vi "DataTXTFileRichInfo.vi"(9 "Language":u32, 11 "file path (dialog if empty)":path caption="文件路径 （空时为对话框）") -> (0 "路径输出":path, 1 "FileInfo":string, 2 "文件类型":string)   [LabVIEW 2015]
uses:
  <vilib>/regexp/Match Regular Expression.xnode
panel:
  out "匹配子字符串":string
  out "输出 2":string
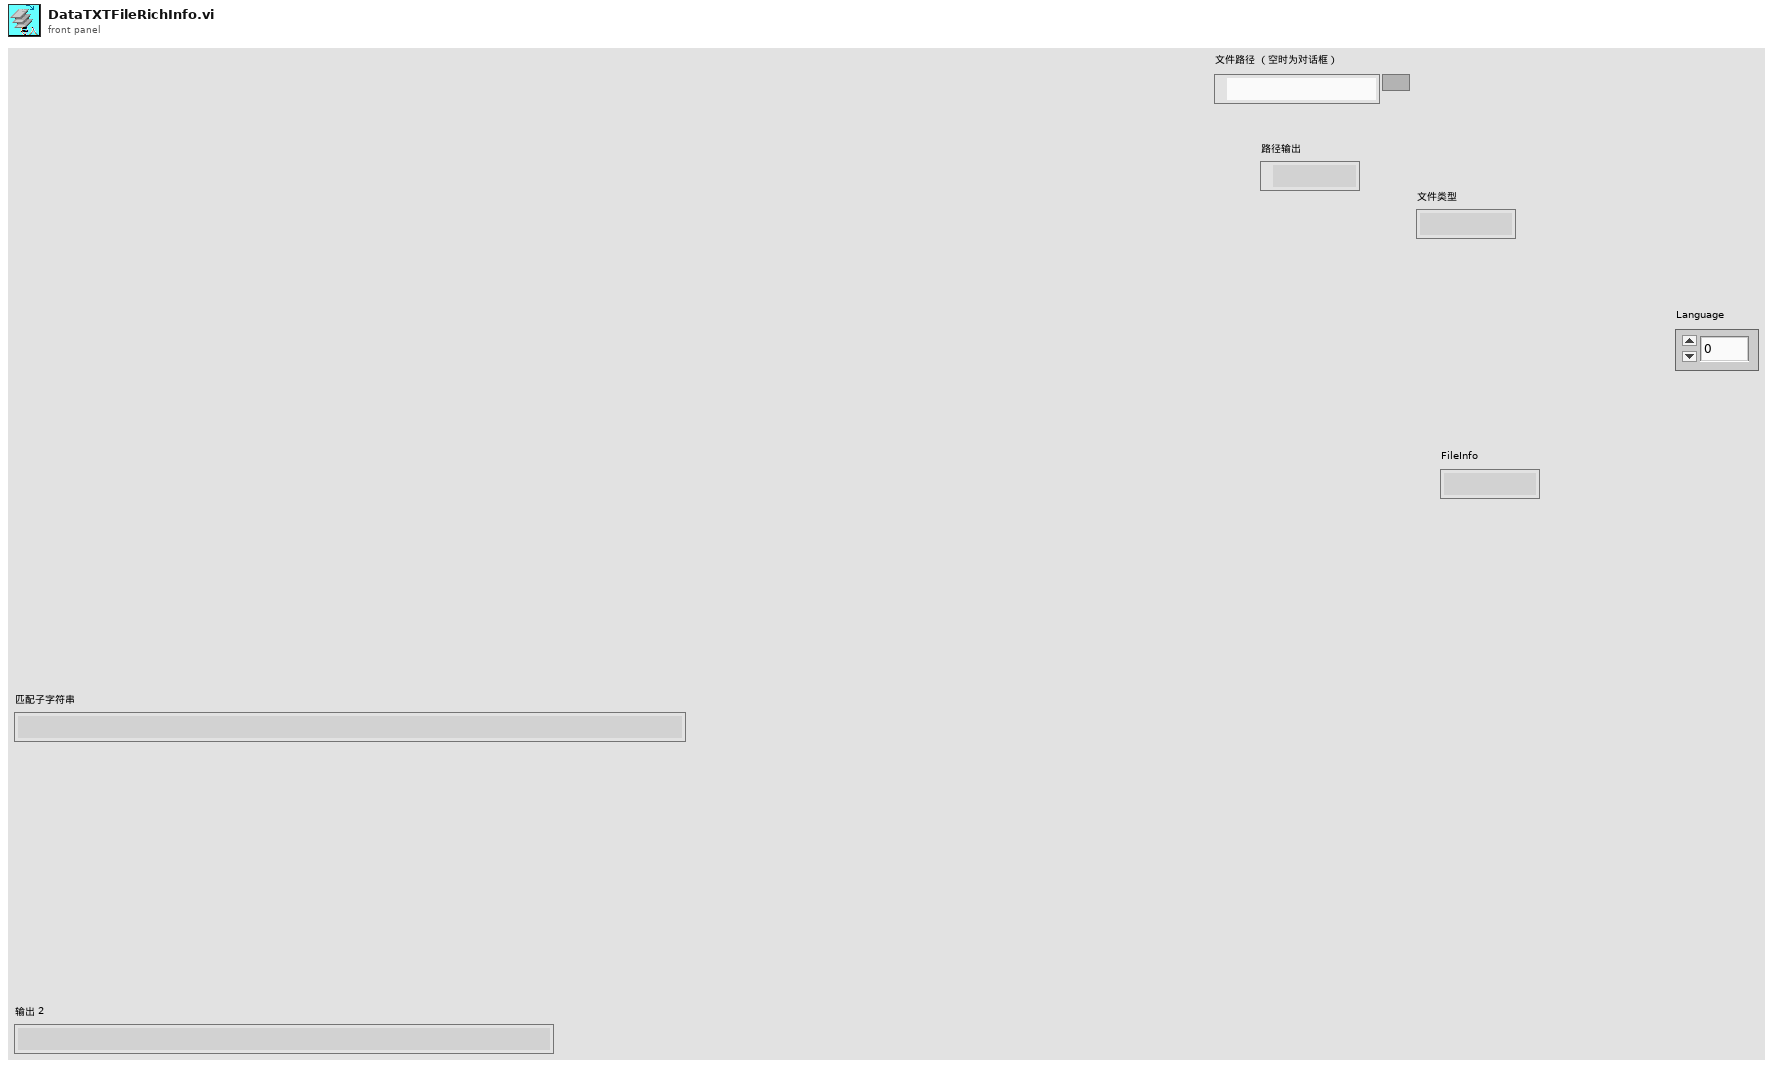
[diagram p1: front panel]
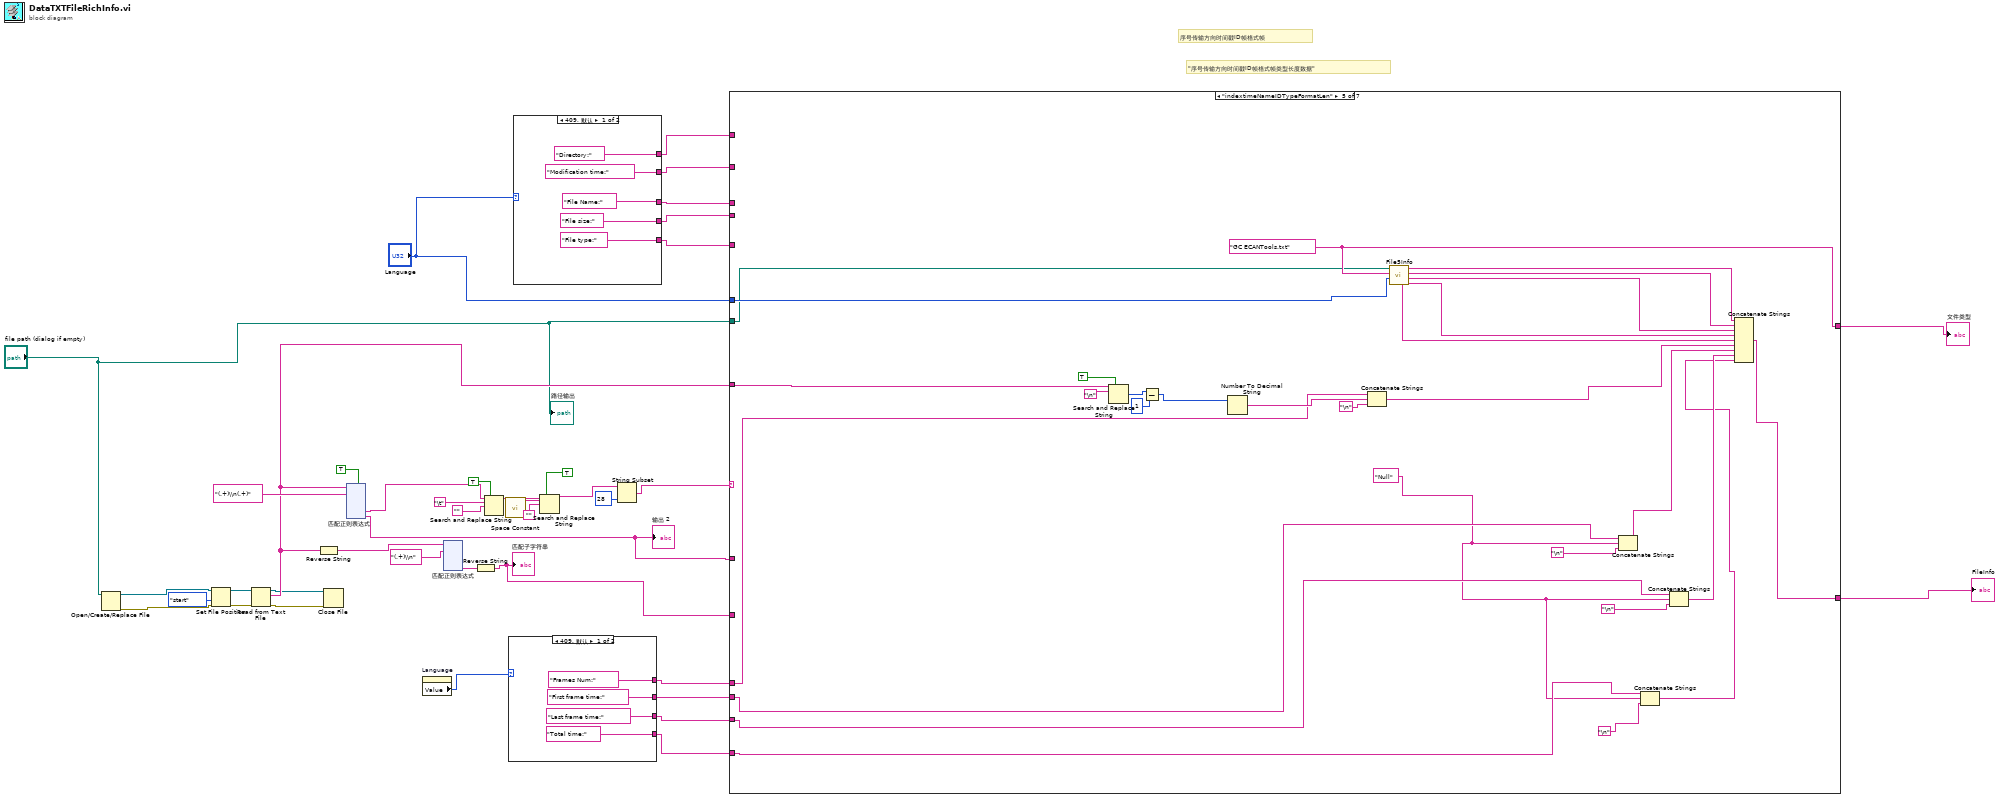
[diagram p0: block diagram]
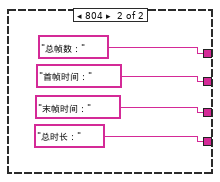
[diagram p2: hidden frame]
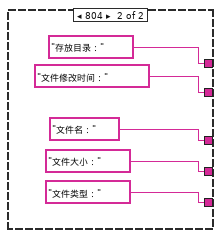
[diagram p3: hidden frame]
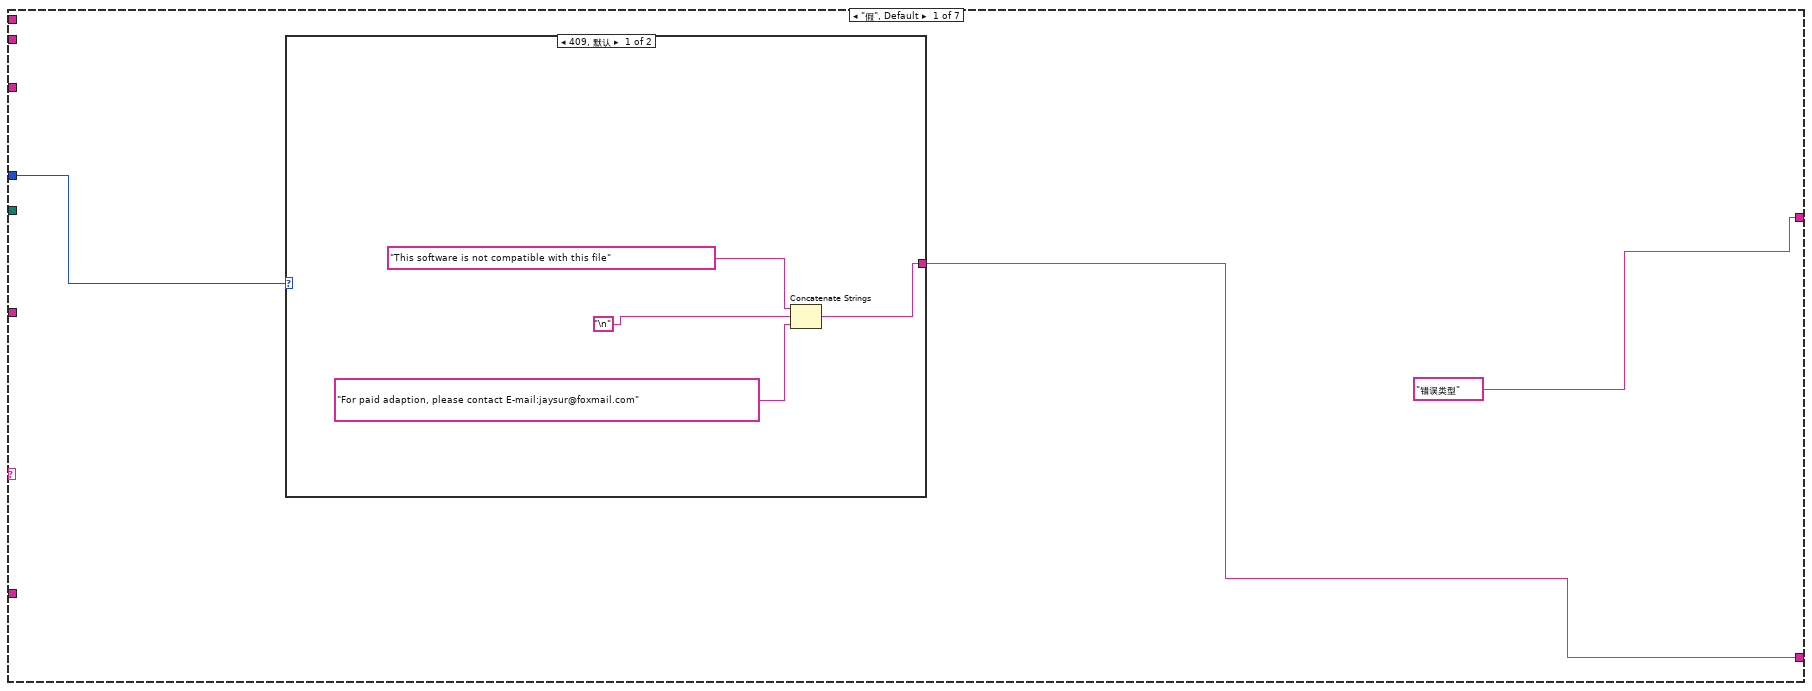
[diagram p4: hidden frame]
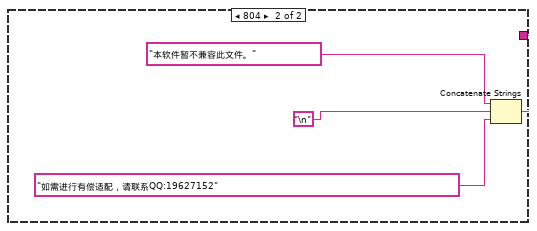
[diagram p5: hidden frame]
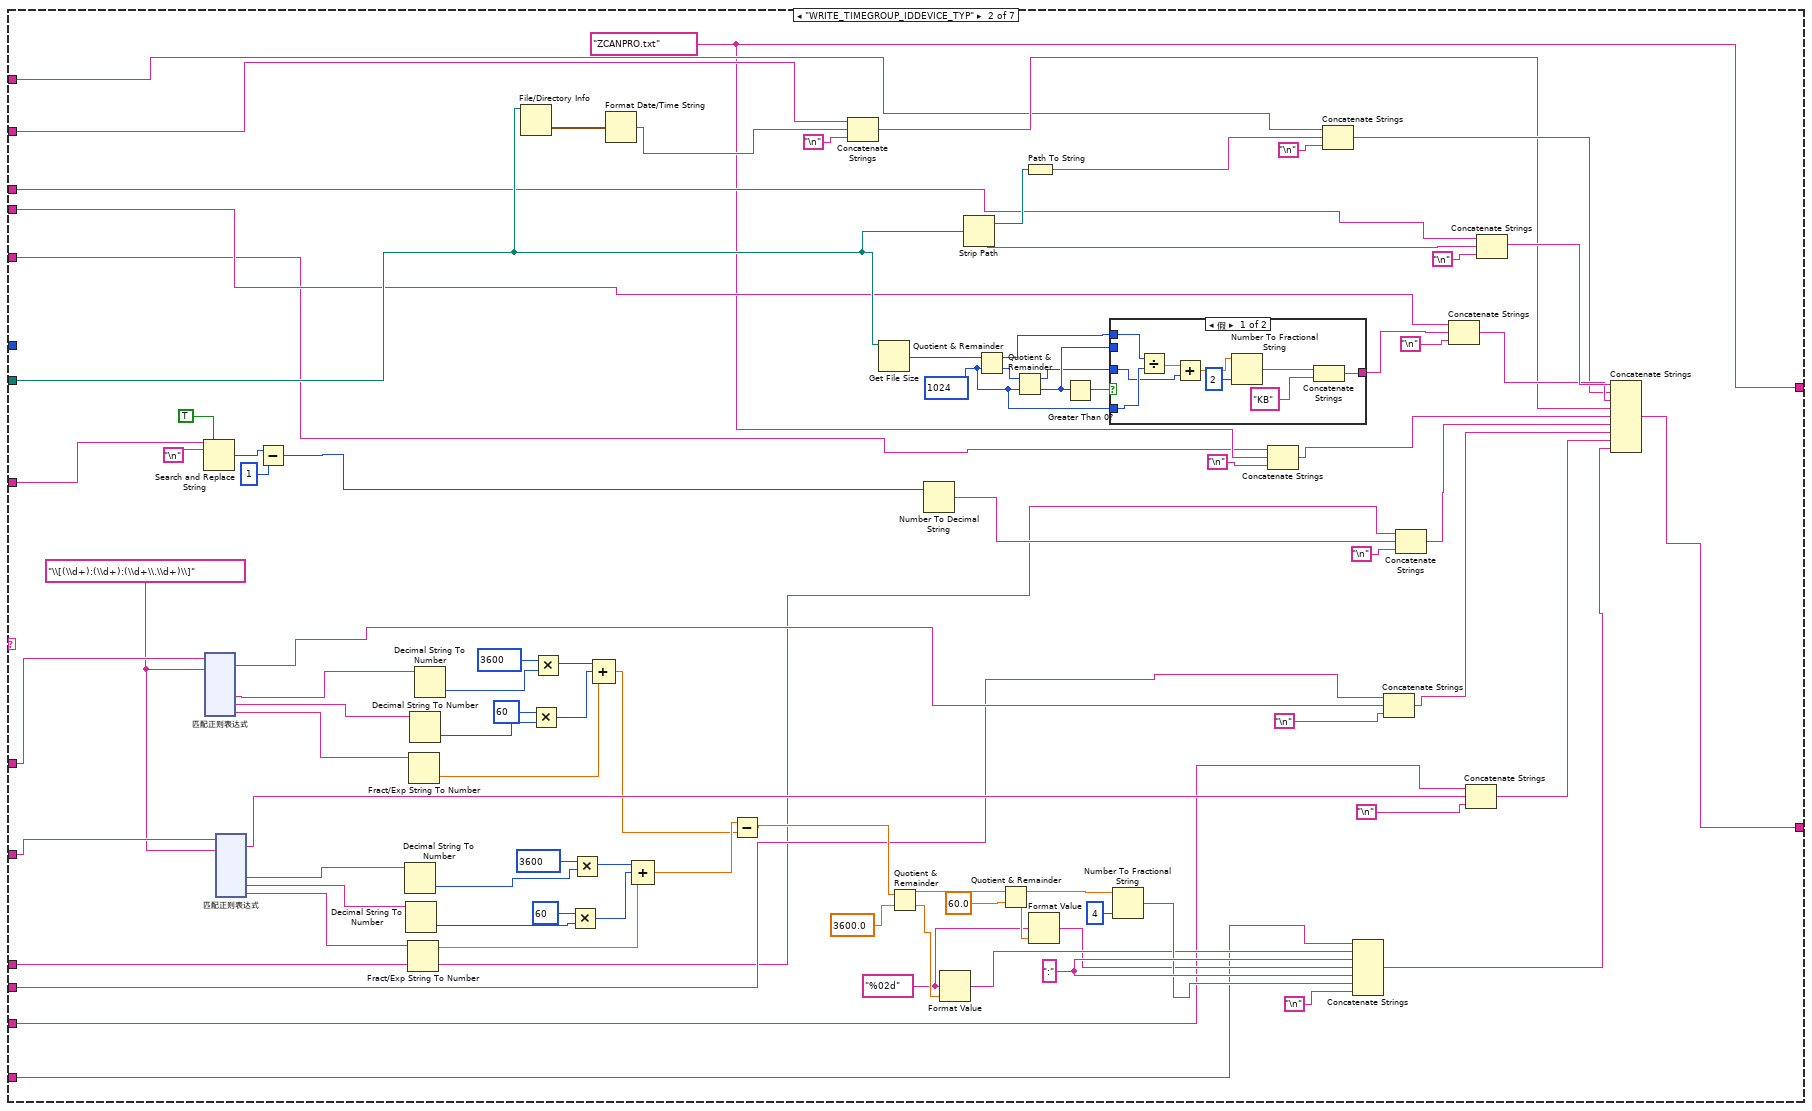
[diagram p6: hidden frame]
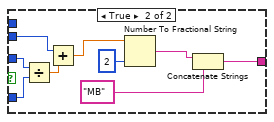
[diagram p7: hidden frame]
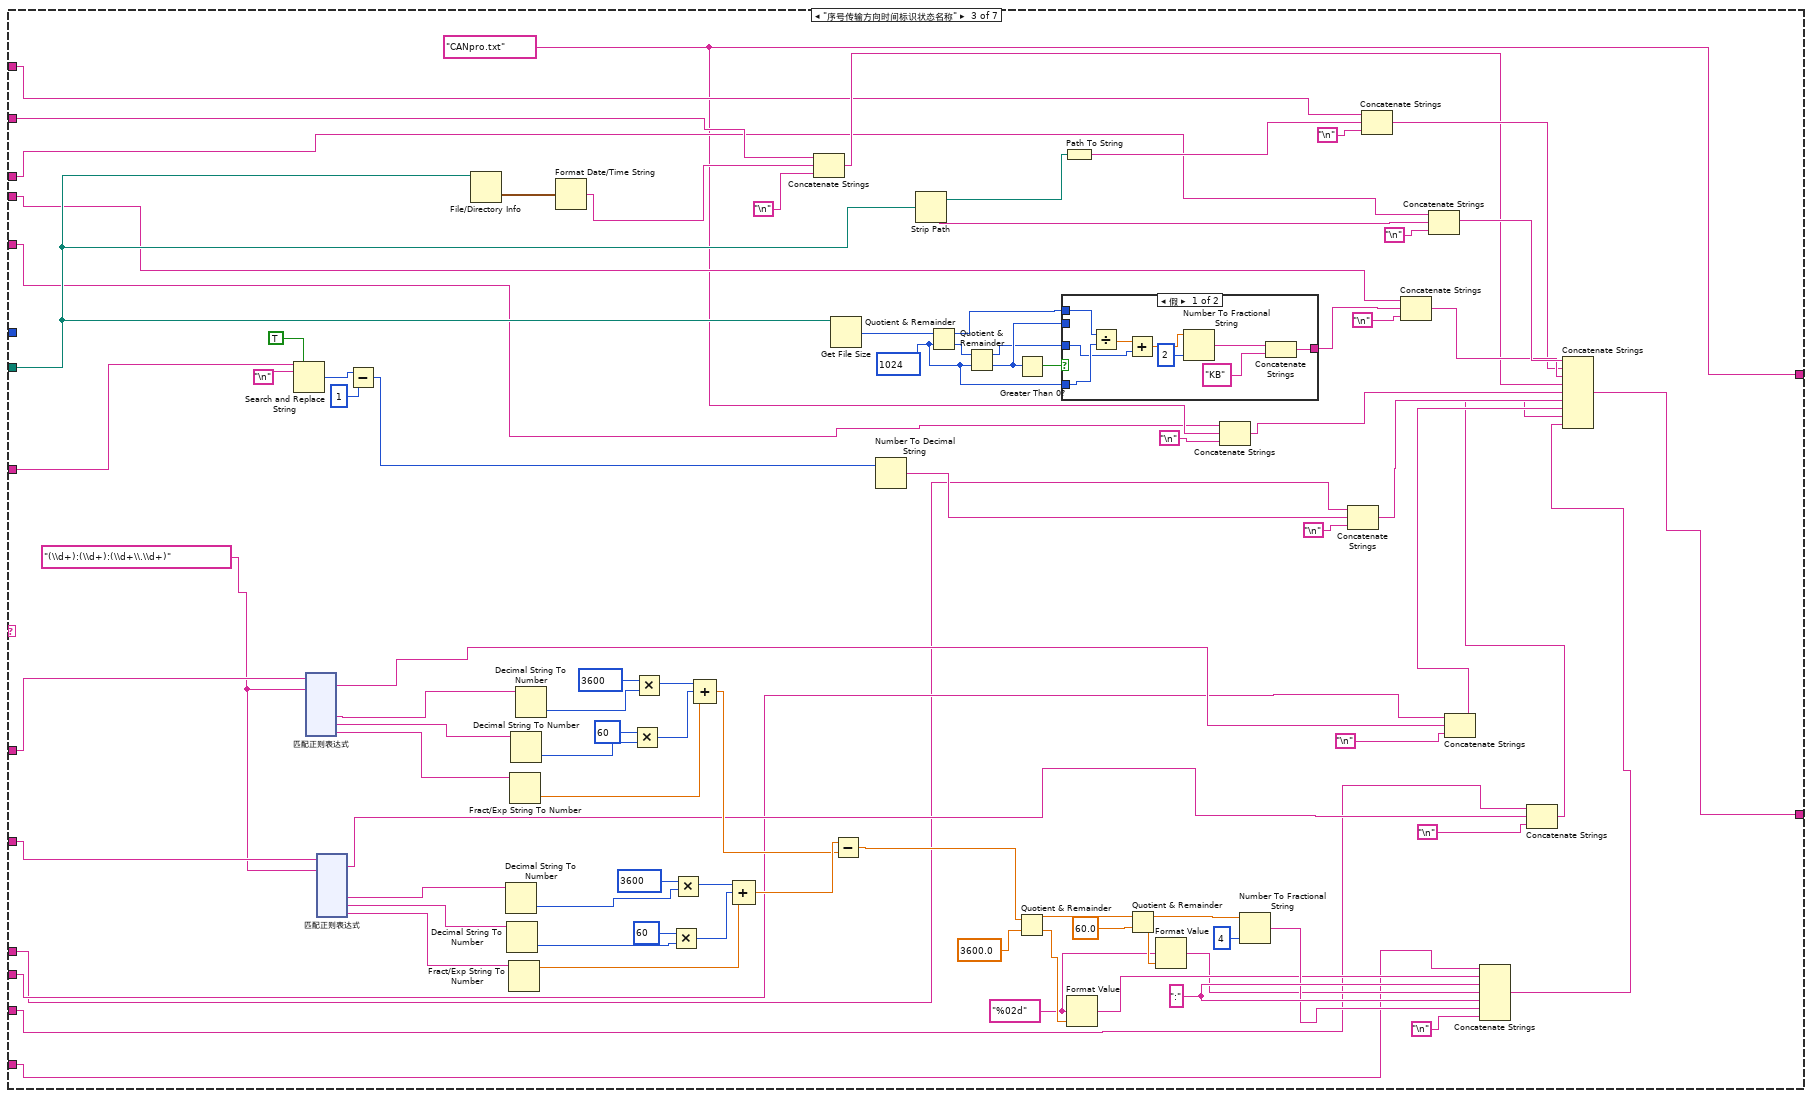
[diagram p8: hidden frame]
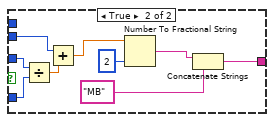
[diagram p9: hidden frame]
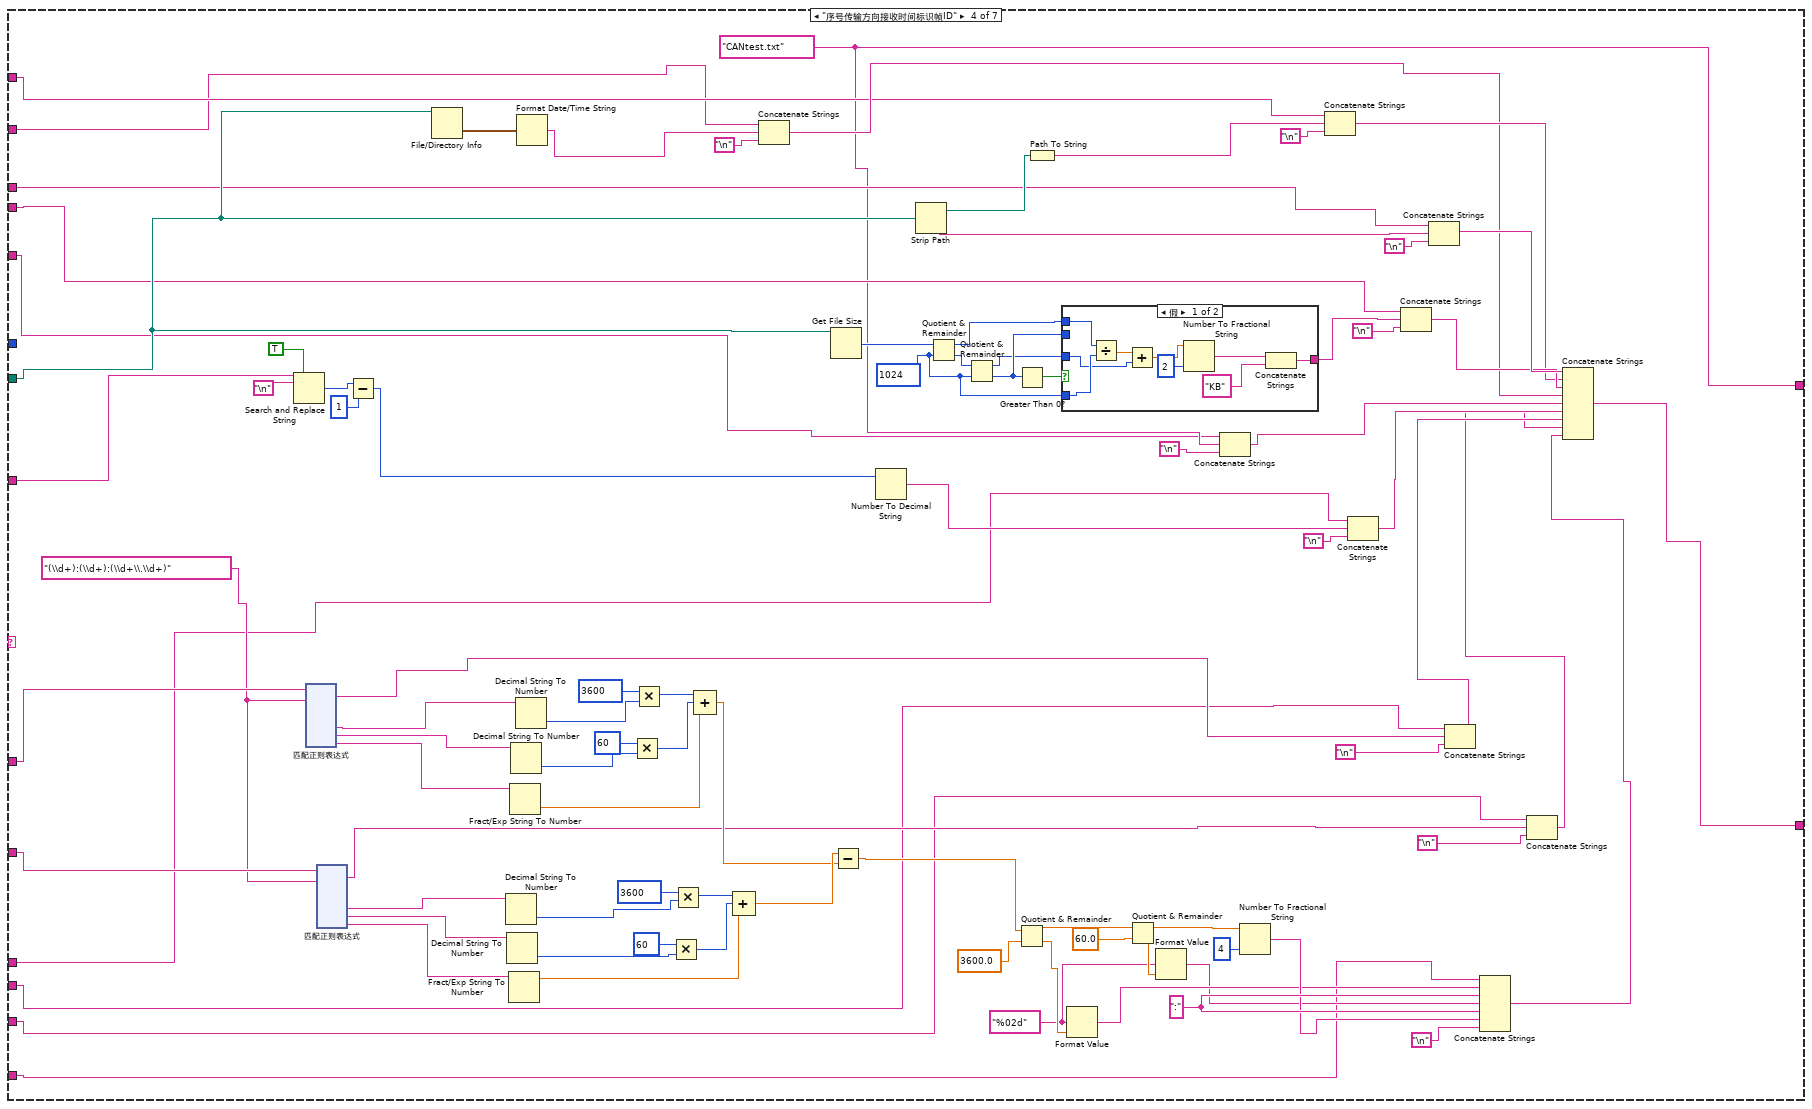
[diagram p10: hidden frame]
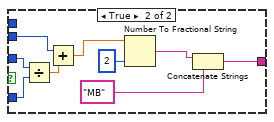
[diagram p11: hidden frame]
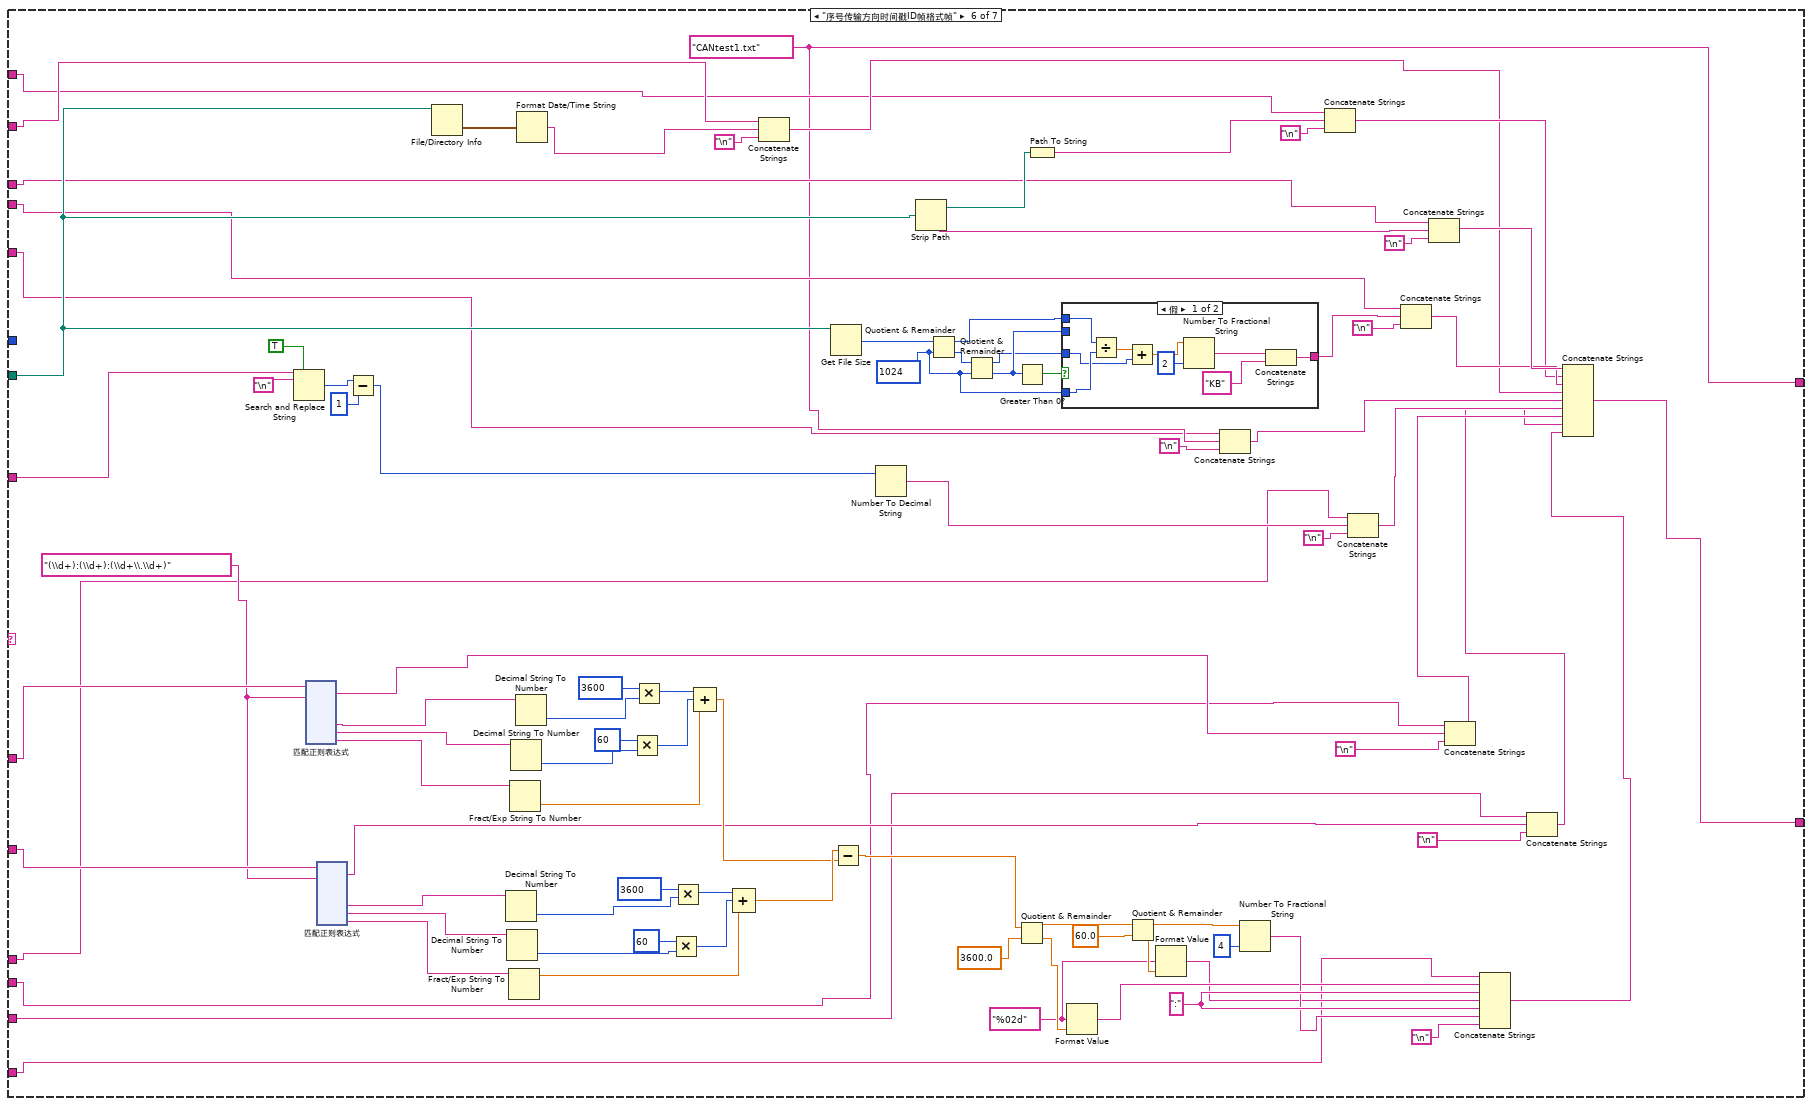
[diagram p12: hidden frame]
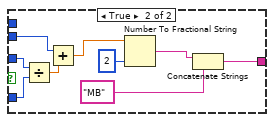
[diagram p13: hidden frame]
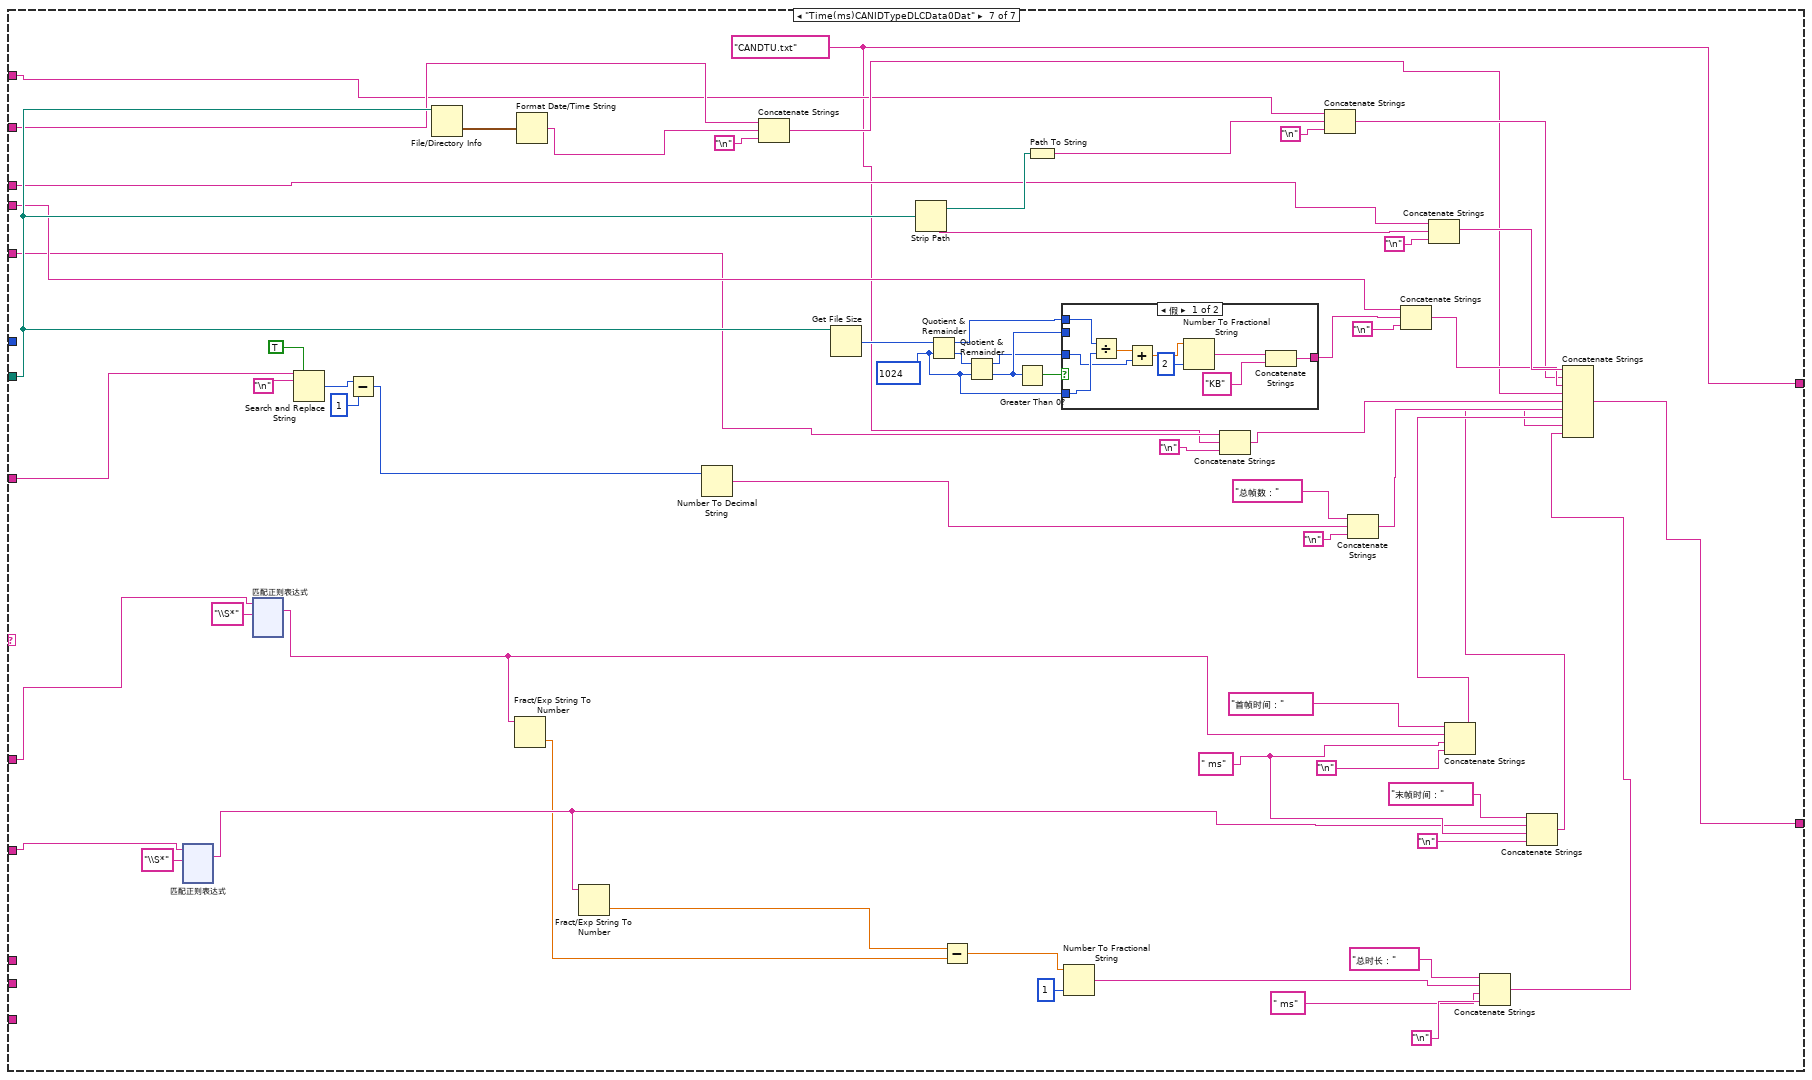
[diagram p14: hidden frame]
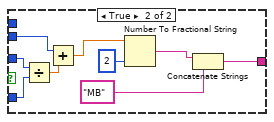
[diagram p15: hidden frame]
diagram:
  # "序号传输方向时间戳ID帧格式帧"
  # "\"序号传输方向时间戳ID帧格式帧类型长度数据\""
  n1 = Open/Create/Replace File(file path (use dialog)="file path (dialog if empty)") -> (refnum out=w17:refnum<file>, error out=w16:errorcluster)  [unwired: 5 in, 1 out]
  n2 = Set File Position(refnum=w17, from (0:start)=enum16{"start", "end", "current"}."start" ("自（0:起始）"), error in=w16) -> (refnum out=w38:refnum<file>, error out=w36:errorcluster)  [unwired: 1 in]
  n3 = Read from Text File(file (use dialog)=w38, error in=w36) -> (refnum out=w14:refnum<file>, text=w20:string, error out=w15:errorcluster)  [unwired: 2 in, 1 out]
  n4 = Reverse String(1:w20) -> (0:w24:string)
  n5 = Close File(refnum=w14, error in=w15) -> ()  [unwired: 2 out]
  n6 = xnode "匹配正则表达式"("输入字符串"=w20, "正则表达式"="(.+)\\n(.+)", "多行？(F)"=TRUE) -> ("子匹配 1"=w31:string, "子匹配 2"=w18:string)  [unwired: 3 in, 5 out]
  "输出 2" <- w18
  n7 = property on="Language" class="DigNum (严格)"() -> ("Value"=w10:u32)  [unwired: 2 in, 2 out]
  n8 = xnode "匹配正则表达式"("输入字符串"=w24, "正则表达式"="(.+)\\n") -> ("子匹配 1"=w23:string)  [unwired: 4 in, 5 out]
  n9 = Reverse String(1:w23) -> (0:w12:string)
  "匹配子字符串" <- w12
  n10 = Search and Replace String(replace all?=TRUE ("替换全部？(F)"), input string=w31, search string="\t", replace string="") -> (result string=w29:string)  [unwired: 4 in, 3 out]
  n11 = call <vilib>:"Space Constant.vi"() -> ("String"=w28:string)
  n12 = case shown="409, 默认" w10 {
    tunnel: ["Total time:" "总时长："] -> w1
    tunnel: ["Last frame time:" "末帧时间："] -> w4
    tunnel: ["First frame time:" "首帧时间："] -> w3
    tunnel: ["Frames Num:" "总帧数："] -> w2
    frame 409, Default {
    }
    frame 804 {
    }
  }
  n13 = case shown="409, 默认" "Language" {
    tunnel: ["Modification time:" "文件修改时间："] -> w9
    tunnel: ["Directory:" "存放目录："] -> w8
    tunnel: ["File Name:" "文件名："] -> w7
    tunnel: ["File size:" "文件大小："] -> w6
    tunnel: ["File type:" "文件类型："] -> w5
    frame 409, Default {
    }
    frame 804 {
    }
  }
  n14 = Search and Replace String(replace all?=TRUE ("替换全部？(F)"), input string=w29, search string=w28, replace string="") -> (result string=w22:string)  [unwired: 4 in, 3 out]
  n15 = String Subset(string=w22, length (rest)=28 ("长度（剩余）")) -> (substring=w19:string)  [unwired: 1 in]
  n16 = case shown="\"indextimeNameIDTypeFormatLen\"" w19 {
    tunnel: [w60 w126 w467 w811 w1119 w1184 w1509] -> w40
    tunnel: ["错误类型" w75 w419 w763 w1105 w1136 w1475] -> w39
    tunnel: "file path (dialog if empty)" -> [_ w81 w425 w768 w1104 w1141 w1494]
    tunnel: w20 -> [_ w118 w462 w806 w1114 w1179 w1504]
    tunnel: w18 -> [_ w114 w438 w782 _ w1155 w1492]
    tunnel: w12 -> [_ w116 w437 w781 _ w1154 w1490]
    tunnel: "Language" -> [w59 _ _ _ w1106 _ _]
    tunnel: w9 -> [_ w79 w423 w766 _ w1140 w1480]
    tunnel: w8 -> [_ w78 w422 w767 _ w1139 w1479]
    tunnel: w7 -> [_ w77 w421 w765 _ w1138 w1478]
    tunnel: w6 -> [_ w76 w420 w764 _ w1137 w1477]
    tunnel: w5 -> [_ w74 w418 w762 _ w1135 w1476]
    tunnel: w1 -> [_ w73 w417 w761 w1110 w1134 _]
    tunnel: w4 -> [_ w72 w416 w760 w1109 w1133 _]
    tunnel: w3 -> [_ w71 w415 w759 w1108 w1132 _]
    tunnel: w2 -> [_ w70 w414 w758 w1107 w1131 _]
    frame "假", Default {
      n17 = case shown="409, 默认" w59 {
        tunnel: [w62 w66] -> w60
        frame 409, Default {
          n18 = Concatenate Strings("This software is not compatible with this file", "\n", "For paid adaption, please contact E-mail:jaysur@foxmail.com") -> (w62:string)
        }
        frame 804 {
          n19 = Concatenate Strings("本软件暂不兼容此文件。", "\n", "如需进行有偿适配，请联系QQ:19627152") -> (w66:string)
        }
      }
    }
    frame "WRITE_TIMEGROUP_IDDEVICE_TYP" {
      w113 = "\\[(\\d+):(\\d+):(\\d+\\.\\d+)\\]"
      w131 = i64 1024 ("y")
      w148 = "%02d" ("格式字符串")
      w154 = ":"
      w75 = "ZCANPRO.txt"
      n20 = Search and Replace String(replace all?=TRUE ("替换全部？(F)"), input string=w118, search string="\n") -> (number of replacements=w120:i32)  [unwired: 5 in, 3 out]
      n21 = xnode "匹配正则表达式"("输入字符串"=w114, "正则表达式"=w113) -> ("所有匹配"=w112:string, "子匹配 1"=w111:string, "子匹配 2"=w110:string, "子匹配 3"=w109:string)  [unwired: 4 in, 4 out]
      n22 = xnode "匹配正则表达式"("输入字符串"=w116, "正则表达式"=w113) -> ("所有匹配"=w115:string, "子匹配 1"=w108:string, "子匹配 2"=w107:string, "子匹配 3"=w106:string)  [unwired: 4 in, 4 out]
      n23 = Subtract(x=w120, y=1) -> (x-y=w117:i32)
      n24 = Decimal String To Number(string=w108) -> (number=w94:i32)  [unwired: 2 in, 1 out]
      n25 = Decimal String To Number(string=w107) -> (number=w93:i32)  [unwired: 2 in, 1 out]
      n26 = Fract/Exp String To Number(string=w106) -> (number=w92:dbl)  [unwired: 3 in, 1 out]
      n27 = Fract/Exp String To Number(string=w109) -> (number=w99:dbl)  [unwired: 3 in, 1 out]
      n28 = Decimal String To Number(string=w110) -> (number=w105:i32)  [unwired: 2 in, 1 out]
      n29 = Decimal String To Number(string=w111) -> (number=w103:i32)  [unwired: 2 in, 1 out]
      n30 = File/Directory Info(path=w81) -> (last mod=w84:timestamp)  [unwired: 1 in, 6 out]
      n31 = Multiply(x=60, y=w105) -> (x*y=w100:i32)
      n32 = Multiply(x=3600, y=w103) -> (x*y=w101:i32)
      n33 = Multiply(x=60, y=w93) -> (x*y=w95:i32)
      n34 = Multiply(x=3600, y=w94) -> (x*y=w96:i32)
      n35 = Compound Arithmetic op=ADD(w101, w100, w99) -> (w90:dbl)
      n36 = Format Date/Time String(seconds (now)=w84) -> (date/time string=w82:string)  [unwired: 2 in]
      n37 = Compound Arithmetic op=ADD(w96, w95, w92) -> (w91:dbl)
      n38 = Subtract(x=w91, y=w90) -> (x-y=w89:dbl)
      n39 = Concatenate Strings(w79, w82, "\n") -> (w80:string)
      n40 = Get File Size(file=w81) -> (size (in bytes)=w134:i64)  [unwired: 1 in, 2 out]
      n41 = Quotient & Remainder(x=w89, y=3600.0) -> (x-y*floor(x/y)=w158:dbl, floor(x/y)=w151:dbl)
      n42 = Number To Decimal String(number=w117) -> (decimal integer string=w137:string)  [unwired: 1 in]
      n43 = Format Value(format string=w148, value (0)=w151) -> (output string=w152:string)  [unwired: 1 in]
      n44 = Strip Path(path=w81) -> (stripped path=w86:path, name=w144:string)
      n45 = Quotient & Remainder(x=w134, y=w131) -> (x-y*floor(x/y)=w127:i64, floor(x/y)=w133:i64)
      n46 = Quotient & Remainder(x=w158, y=60.0) -> (x-y*floor(x/y)=w156:dbl, floor(x/y)=w150:dbl)
      n47 = Quotient & Remainder(x=w133, y=w131) -> (x-y*floor(x/y)=w129:i64, floor(x/y)=w130:i64)
      n48 = Path To String(path=w86) -> (string=w87:string)
      n49 = Format Value(format string=w148, value (0)=w150) -> (output string=w149:string)  [unwired: 1 in]
      n50 = Greater Than 0?(x=w130) -> (x > 0?=w132:bool)
      n51 = case shown="假" w132 {
        tunnel: w131 -> [w401 w411]
        tunnel: w130 -> [_ w409]
        tunnel: w129 -> [w399 w412]
        tunnel: [w404 w407] -> w128
        tunnel: w127 -> [w402 _]
        frame False {
          n52 = Divide(x=w402, y=w401) -> (x/y=w400:dbl)
          n53 = Add(x=w400, y=w399) -> (x+y=w398:dbl)
          n54 = Number To Fractional String(number=w398, precision (6)=i16 2 ("精度(6)")) -> (F-format string=w396:string)  [unwired: 2 in]
          n55 = Concatenate Strings(w396, "KB" ("字符串")) -> (w404:string)
        }
        frame True {
          n56 = Divide(x=w412, y=w411) -> (x/y=w410:dbl)
          n57 = Add(x=w409, y=w410) -> (x+y=w408:dbl)
          n58 = Number To Fractional String(number=w408, precision (6)=i16 2 ("精度(6)")) -> (F-format string=w406:string)  [unwired: 2 in]
          n59 = Concatenate Strings(w406, "MB") -> (w407:string)
        }
      }
      n60 = Number To Fractional String(number=w156, precision (6)=i16 4 ("精度(6)")) -> (F-format string=w153:string)  [unwired: 2 in]
      n61 = Concatenate Strings(w74, w75, "\n") -> (w141:string)
      n62 = Concatenate Strings(w78, w87, "\n") -> (w85:string)
      n63 = Concatenate Strings(w73, w152, w154, w149, w154, w153, "\n") -> (w125:string)
      n64 = Concatenate Strings(w71, w112, "\n") -> (w123:string)
      n65 = Concatenate Strings(w70, w137, "\n") -> (w138:string)
      n66 = Concatenate Strings(w76, w128, "\n") -> (w135:string)
      n67 = Concatenate Strings(w72, w115, "\n") -> (w124:string)
      n68 = Concatenate Strings(w77, w144, "\n") -> (w143:string)
      n69 = Concatenate Strings(w143, w85, w135, w80, w141, w138, w123, w124, w125) -> (w126:string)
    }
    frame "序号传输方向时间标识状态名称" {
      w434 = "(\\d+):(\\d+):(\\d+\\.\\d+)"
      w475 = i64 1024 ("y")
      w492 = "%02d" ("格式字符串")
      w498 = ":"
      w419 = "CANpro.txt"
      n70 = Search and Replace String(replace all?=TRUE ("替换全部？(F)"), input string=w462, search string="\n") -> (number of replacements=w464:i32)  [unwired: 5 in, 3 out]
      n71 = xnode "匹配正则表达式"("输入字符串"=w438, "正则表达式"=w434) -> ("所有匹配"=w436:string, "子匹配 1"=w460:string, "子匹配 2"=w459:string, "子匹配 3"=w458:string)  [unwired: 4 in, 4 out]
      n72 = xnode "匹配正则表达式"("输入字符串"=w437, "正则表达式"=w434) -> ("所有匹配"=w435:string, "子匹配 1"=w457:string, "子匹配 2"=w456:string, "子匹配 3"=w455:string)  [unwired: 4 in, 4 out]
      n73 = Subtract(x=w464, y=1) -> (x-y=w461:i32)
      n74 = File/Directory Info(path=w425) -> (last mod=w428:timestamp)  [unwired: 1 in, 6 out]
      n75 = Decimal String To Number(string=w457) -> (number=w443:i32)  [unwired: 2 in, 1 out]
      n76 = Decimal String To Number(string=w456) -> (number=w442:i32)  [unwired: 2 in, 1 out]
      n77 = Fract/Exp String To Number(string=w455) -> (number=w441:dbl)  [unwired: 3 in, 1 out]
      n78 = Fract/Exp String To Number(string=w458) -> (number=w448:dbl)  [unwired: 3 in, 1 out]
      n79 = Decimal String To Number(string=w459) -> (number=w454:i32)  [unwired: 2 in, 1 out]
      n80 = Decimal String To Number(string=w460) -> (number=w452:i32)  [unwired: 2 in, 1 out]
      n81 = Format Date/Time String(seconds (now)=w428) -> (date/time string=w426:string)  [unwired: 2 in]
      n82 = Multiply(x=60, y=w454) -> (x*y=w449:i32)
      n83 = Multiply(x=3600, y=w452) -> (x*y=w450:i32)
      n84 = Multiply(x=60, y=w442) -> (x*y=w444:i32)
      n85 = Multiply(x=3600, y=w443) -> (x*y=w445:i32)
      n86 = Compound Arithmetic op=ADD(w450, w449, w448) -> (w439:dbl)
      n87 = Compound Arithmetic op=ADD(w445, w444, w441) -> (w440:dbl)
      n88 = Concatenate Strings(w423, w426, "\n") -> (w424:string)
      n89 = Get File Size(file=w425) -> (size (in bytes)=w478:i64)  [unwired: 1 in, 2 out]
      n90 = Subtract(x=w440, y=w439) -> (x-y=w433:dbl)
      n91 = Number To Decimal String(number=w461) -> (decimal integer string=w481:string)  [unwired: 1 in]
      n92 = Strip Path(path=w425) -> (stripped path=w430:path, name=w488:string)
      n93 = Quotient & Remainder(x=w478, y=w475) -> (x-y*floor(x/y)=w471:i64, floor(x/y)=w477:i64)
      n94 = Quotient & Remainder(x=w477, y=w475) -> (x-y*floor(x/y)=w473:i64, floor(x/y)=w474:i64)
      n95 = Greater Than 0?(x=w474) -> (x > 0?=w476:bool)
      n96 = Quotient & Remainder(x=w433, y=3600.0) -> (x-y*floor(x/y)=w502:dbl, floor(x/y)=w495:dbl)
      n97 = case shown="假" w476 {
        tunnel: w475 -> [w745 w755]
        tunnel: w474 -> [_ w753]
        tunnel: w473 -> [w743 w756]
        tunnel: [w748 w751] -> w472
        tunnel: w471 -> [w746 _]
        frame False {
          n98 = Divide(x=w746, y=w745) -> (x/y=w744:dbl)
          n99 = Add(x=w744, y=w743) -> (x+y=w742:dbl)
          n100 = Number To Fractional String(number=w742, precision (6)=i16 2 ("精度(6)")) -> (F-format string=w740:string)  [unwired: 2 in]
          n101 = Concatenate Strings(w740, "KB" ("字符串")) -> (w748:string)
        }
        frame True {
          n102 = Divide(x=w756, y=w755) -> (x/y=w754:dbl)
          n103 = Add(x=w753, y=w754) -> (x+y=w752:dbl)
          n104 = Number To Fractional String(number=w752, precision (6)=i16 2 ("精度(6)")) -> (F-format string=w750:string)  [unwired: 2 in]
          n105 = Concatenate Strings(w750, "MB") -> (w751:string)
        }
      }
      n106 = Path To String(path=w430) -> (string=w431:string)
      n107 = Format Value(format string=w492, value (0)=w495) -> (output string=w496:string)  [unwired: 1 in]
      n108 = Quotient & Remainder(x=w502, y=60.0) -> (x-y*floor(x/y)=w500:dbl, floor(x/y)=w494:dbl)
      n109 = Format Value(format string=w492, value (0)=w494) -> (output string=w493:string)  [unwired: 1 in]
      n110 = Concatenate Strings(w418, w419, "\n") -> (w485:string)
      n111 = Number To Fractional String(number=w500, precision (6)=i16 4 ("精度(6)")) -> (F-format string=w497:string)  [unwired: 2 in]
      n112 = Concatenate Strings(w414, w481, "\n") -> (w482:string)
      n113 = Concatenate Strings(w422, w431, "\n") -> (w429:string)
      n114 = Concatenate Strings(w420, w472, "\n") -> (w479:string)
      n115 = Concatenate Strings(w421, w488, "\n") -> (w487:string)
      n116 = Concatenate Strings(w415, w436, "\n") -> (w470:string)
      n117 = Concatenate Strings(w417, w496, w498, w493, w498, w497, "\n") -> (w468:string)
      n118 = Concatenate Strings(w416, w435, "\n") -> (w469:string)
      n119 = Concatenate Strings(w487, w429, w479, w424, w485, w482, w470, w469, w468) -> (w467:string)
    }
    frame "序号传输方向接收时间标识帧ID" {
      w778 = "(\\d+):(\\d+):(\\d+\\.\\d+)"
      w819 = i64 1024 ("y")
      w836 = "%02d" ("格式字符串")
      w842 = ":"
      w763 = "CANtest.txt"
      n120 = Search and Replace String(replace all?=TRUE ("替换全部？(F)"), input string=w806, search string="\n") -> (number of replacements=w808:i32)  [unwired: 5 in, 3 out]
      n121 = xnode "匹配正则表达式"("输入字符串"=w782, "正则表达式"=w778) -> ("所有匹配"=w780:string, "子匹配 1"=w804:string, "子匹配 2"=w803:string, "子匹配 3"=w802:string)  [unwired: 4 in, 4 out]
      n122 = xnode "匹配正则表达式"("输入字符串"=w781, "正则表达式"=w778) -> ("所有匹配"=w779:string, "子匹配 1"=w801:string, "子匹配 2"=w800:string, "子匹配 3"=w799:string)  [unwired: 4 in, 4 out]
      n123 = Subtract(x=w808, y=1) -> (x-y=w805:i32)
      n124 = File/Directory Info(path=w768) -> (last mod=w772:timestamp)  [unwired: 1 in, 6 out]
      n125 = Decimal String To Number(string=w801) -> (number=w787:i32)  [unwired: 2 in, 1 out]
      n126 = Decimal String To Number(string=w800) -> (number=w786:i32)  [unwired: 2 in, 1 out]
      n127 = Fract/Exp String To Number(string=w799) -> (number=w785:dbl)  [unwired: 3 in, 1 out]
      n128 = Fract/Exp String To Number(string=w802) -> (number=w792:dbl)  [unwired: 3 in, 1 out]
      n129 = Decimal String To Number(string=w803) -> (number=w798:i32)  [unwired: 2 in, 1 out]
      n130 = Decimal String To Number(string=w804) -> (number=w796:i32)  [unwired: 2 in, 1 out]
      n131 = Format Date/Time String(seconds (now)=w772) -> (date/time string=w770:string)  [unwired: 2 in]
      n132 = Multiply(x=60, y=w798) -> (x*y=w793:i32)
      n133 = Multiply(x=3600, y=w796) -> (x*y=w794:i32)
      n134 = Multiply(x=60, y=w786) -> (x*y=w788:i32)
      n135 = Multiply(x=3600, y=w787) -> (x*y=w789:i32)
      n136 = Compound Arithmetic op=ADD(w794, w793, w792) -> (w783:dbl)
      n137 = Compound Arithmetic op=ADD(w789, w788, w785) -> (w784:dbl)
      n138 = Concatenate Strings(w766, w770, "\n") -> (w769:string)
      n139 = Get File Size(file=w768) -> (size (in bytes)=w822:i64)  [unwired: 1 in, 2 out]
      n140 = Subtract(x=w784, y=w783) -> (x-y=w777:dbl)
      n141 = Number To Decimal String(number=w805) -> (decimal integer string=w825:string)  [unwired: 1 in]
      n142 = Strip Path(path=w768) -> (stripped path=w774:path, name=w832:string)
      n143 = Quotient & Remainder(x=w822, y=w819) -> (x-y*floor(x/y)=w815:i64, floor(x/y)=w821:i64)
      n144 = Quotient & Remainder(x=w821, y=w819) -> (x-y*floor(x/y)=w817:i64, floor(x/y)=w818:i64)
      n145 = Greater Than 0?(x=w818) -> (x > 0?=w820:bool)
      n146 = Quotient & Remainder(x=w777, y=3600.0) -> (x-y*floor(x/y)=w846:dbl, floor(x/y)=w839:dbl)
      n147 = Path To String(path=w774) -> (string=w775:string)
      n148 = case shown="假" w820 {
        tunnel: w819 -> [w1089 w1099]
        tunnel: w818 -> [_ w1097]
        tunnel: w817 -> [w1087 w1100]
        tunnel: [w1092 w1095] -> w816
        tunnel: w815 -> [w1090 _]
        frame False {
          n149 = Divide(x=w1090, y=w1089) -> (x/y=w1088:dbl)
          n150 = Add(x=w1088, y=w1087) -> (x+y=w1086:dbl)
          n151 = Number To Fractional String(number=w1086, precision (6)=i16 2 ("精度(6)")) -> (F-format string=w1084:string)  [unwired: 2 in]
          n152 = Concatenate Strings(w1084, "KB" ("字符串")) -> (w1092:string)
        }
        frame True {
          n153 = Divide(x=w1100, y=w1099) -> (x/y=w1098:dbl)
          n154 = Add(x=w1097, y=w1098) -> (x+y=w1096:dbl)
          n155 = Number To Fractional String(number=w1096, precision (6)=i16 2 ("精度(6)")) -> (F-format string=w1094:string)  [unwired: 2 in]
          n156 = Concatenate Strings(w1094, "MB") -> (w1095:string)
        }
      }
      n157 = Format Value(format string=w836, value (0)=w839) -> (output string=w840:string)  [unwired: 1 in]
      n158 = Quotient & Remainder(x=w846, y=60.0) -> (x-y*floor(x/y)=w844:dbl, floor(x/y)=w838:dbl)
      n159 = Format Value(format string=w836, value (0)=w838) -> (output string=w837:string)  [unwired: 1 in]
      n160 = Concatenate Strings(w762, w763, "\n") -> (w829:string)
      n161 = Number To Fractional String(number=w844, precision (6)=i16 4 ("精度(6)")) -> (F-format string=w841:string)  [unwired: 2 in]
      n162 = Concatenate Strings(w767, w775, "\n") -> (w773:string)
      n163 = Concatenate Strings(w758, w825, "\n") -> (w826:string)
      n164 = Concatenate Strings(w764, w816, "\n") -> (w823:string)
      n165 = Concatenate Strings(w765, w832, "\n") -> (w831:string)
      n166 = Concatenate Strings(w759, w780, "\n") -> (w814:string)
      n167 = Concatenate Strings(w761, w840, w842, w837, w842, w841, "\n") -> (w812:string)
      n168 = Concatenate Strings(w760, w779, "\n") -> (w813:string)
      n169 = Concatenate Strings(w831, w773, w823, w769, w829, w826, w814, w813, w812) -> (w811:string)
    }
    frame "indextimeNameIDTypeFormatLen" {
      w1103 = "Null"
      w1105 = "GC ECANTools.txt"
      n170 = Search and Replace String(replace all?=TRUE ("替换全部？(F)"), input string=w1114, search string="\n") -> (number of replacements=w1116:i32)  [unwired: 5 in, 3 out]
      n171 = Subtract(x=w1116, y=1) -> (x-y=w1113:i32)
      n172 = Number To Decimal String(number=w1113) -> (decimal integer string=w1124:string)  [unwired: 1 in]
      n173 = Concatenate Strings(w1107, w1124, "\n") -> (w1125:string)
      n174 = call "File5Info.vi"("Language"=w1106, "TypeIn"=w1105, "file path (dialog if empty)"=w1104) -> ("ModificationTimeOut"=w1111:string, "FileSizeOut"=w1123:string, "DirectoryOut"=w1112:string, "FileNameOut"=w1128:string, "FileTypeOut"=w1127:string)  [unwired: 4 in]
      n175 = Concatenate Strings(w1108, w1103, "\n") -> (w1122:string)
      n176 = Concatenate Strings(w1110, w1103, "\n") -> (w1120:string)
      n177 = Concatenate Strings(w1109, w1103, "\n") -> (w1121:string)
      n178 = Concatenate Strings(w1128, w1112, w1123, w1111, w1127, w1125, w1122, w1121, w1120) -> (w1119:string)
    }
    frame "序号传输方向时间戳ID帧格式帧" {
      w1151 = "(\\d+):(\\d+):(\\d+\\.\\d+)"
      w1192 = i64 1024 ("y")
      w1209 = "%02d" ("格式字符串")
      w1215 = ":"
      w1136 = "CANtest1.txt"
      n179 = Search and Replace String(replace all?=TRUE ("替换全部？(F)"), input string=w1179, search string="\n") -> (number of replacements=w1181:i32)  [unwired: 5 in, 3 out]
      n180 = xnode "匹配正则表达式"("输入字符串"=w1155, "正则表达式"=w1151) -> ("所有匹配"=w1153:string, "子匹配 1"=w1177:string, "子匹配 2"=w1176:string, "子匹配 3"=w1175:string)  [unwired: 4 in, 4 out]
      n181 = xnode "匹配正则表达式"("输入字符串"=w1154, "正则表达式"=w1151) -> ("所有匹配"=w1152:string, "子匹配 1"=w1174:string, "子匹配 2"=w1173:string, "子匹配 3"=w1172:string)  [unwired: 4 in, 4 out]
      n182 = Subtract(x=w1181, y=1) -> (x-y=w1178:i32)
      n183 = File/Directory Info(path=w1141) -> (last mod=w1145:timestamp)  [unwired: 1 in, 6 out]
      n184 = Decimal String To Number(string=w1174) -> (number=w1160:i32)  [unwired: 2 in, 1 out]
      n185 = Decimal String To Number(string=w1173) -> (number=w1159:i32)  [unwired: 2 in, 1 out]
      n186 = Fract/Exp String To Number(string=w1172) -> (number=w1158:dbl)  [unwired: 3 in, 1 out]
      n187 = Fract/Exp String To Number(string=w1175) -> (number=w1165:dbl)  [unwired: 3 in, 1 out]
      n188 = Decimal String To Number(string=w1176) -> (number=w1171:i32)  [unwired: 2 in, 1 out]
      n189 = Decimal String To Number(string=w1177) -> (number=w1169:i32)  [unwired: 2 in, 1 out]
      n190 = Format Date/Time String(seconds (now)=w1145) -> (date/time string=w1143:string)  [unwired: 2 in]
      n191 = Multiply(x=60, y=w1171) -> (x*y=w1166:i32)
      n192 = Multiply(x=3600, y=w1169) -> (x*y=w1167:i32)
      n193 = Multiply(x=60, y=w1159) -> (x*y=w1161:i32)
      n194 = Multiply(x=3600, y=w1160) -> (x*y=w1162:i32)
      n195 = Compound Arithmetic op=ADD(w1167, w1166, w1165) -> (w1156:dbl)
      n196 = Compound Arithmetic op=ADD(w1162, w1161, w1158) -> (w1157:dbl)
      n197 = Concatenate Strings(w1140, w1143, "\n") -> (w1142:string)
      n198 = Get File Size(file=w1141) -> (size (in bytes)=w1195:i64)  [unwired: 1 in, 2 out]
      n199 = Subtract(x=w1157, y=w1156) -> (x-y=w1150:dbl)
      n200 = Number To Decimal String(number=w1178) -> (decimal integer string=w1198:string)  [unwired: 1 in]
      n201 = Strip Path(path=w1141) -> (stripped path=w1147:path, name=w1205:string)
      n202 = Quotient & Remainder(x=w1195, y=w1192) -> (x-y*floor(x/y)=w1188:i64, floor(x/y)=w1194:i64)
      n203 = Quotient & Remainder(x=w1194, y=w1192) -> (x-y*floor(x/y)=w1190:i64, floor(x/y)=w1191:i64)
      n204 = Greater Than 0?(x=w1191) -> (x > 0?=w1193:bool)
      n205 = Quotient & Remainder(x=w1150, y=3600.0) -> (x-y*floor(x/y)=w1219:dbl, floor(x/y)=w1212:dbl)
      n206 = Path To String(path=w1147) -> (string=w1148:string)
      n207 = case shown="假" w1193 {
        tunnel: w1192 -> [w1462 w1472]
        tunnel: w1191 -> [_ w1470]
        tunnel: w1190 -> [w1460 w1473]
        tunnel: [w1465 w1468] -> w1189
        tunnel: w1188 -> [w1463 _]
        frame False {
          n208 = Divide(x=w1463, y=w1462) -> (x/y=w1461:dbl)
          n209 = Add(x=w1461, y=w1460) -> (x+y=w1459:dbl)
          n210 = Number To Fractional String(number=w1459, precision (6)=i16 2 ("精度(6)")) -> (F-format string=w1457:string)  [unwired: 2 in]
          n211 = Concatenate Strings(w1457, "KB" ("字符串")) -> (w1465:string)
        }
        frame True {
          n212 = Divide(x=w1473, y=w1472) -> (x/y=w1471:dbl)
          n213 = Add(x=w1470, y=w1471) -> (x+y=w1469:dbl)
          n214 = Number To Fractional String(number=w1469, precision (6)=i16 2 ("精度(6)")) -> (F-format string=w1467:string)  [unwired: 2 in]
          n215 = Concatenate Strings(w1467, "MB") -> (w1468:string)
        }
      }
      n216 = Format Value(format string=w1209, value (0)=w1212) -> (output string=w1213:string)  [unwired: 1 in]
      n217 = Quotient & Remainder(x=w1219, y=60.0) -> (x-y*floor(x/y)=w1217:dbl, floor(x/y)=w1211:dbl)
      n218 = Format Value(format string=w1209, value (0)=w1211) -> (output string=w1210:string)  [unwired: 1 in]
      n219 = Concatenate Strings(w1135, w1136, "\n") -> (w1202:string)
      n220 = Number To Fractional String(number=w1217, precision (6)=i16 4 ("精度(6)")) -> (F-format string=w1214:string)  [unwired: 2 in]
      n221 = Concatenate Strings(w1139, w1148, "\n") -> (w1146:string)
      n222 = Concatenate Strings(w1131, w1198, "\n") -> (w1199:string)
      n223 = Concatenate Strings(w1137, w1189, "\n") -> (w1196:string)
      n224 = Concatenate Strings(w1138, w1205, "\n") -> (w1204:string)
      n225 = Concatenate Strings(w1132, w1153, "\n") -> (w1187:string)
      n226 = Concatenate Strings(w1134, w1213, w1215, w1210, w1215, w1214, "\n") -> (w1185:string)
      n227 = Concatenate Strings(w1133, w1152, "\n") -> (w1186:string)
      n228 = Concatenate Strings(w1204, w1146, w1196, w1142, w1202, w1199, w1187, w1186, w1185) -> (w1184:string)
    }
    frame "Time(ms)CANIDTypeDLCData0Dat" {
      w1489 = " ms"
      w1517 = i64 1024 ("y")
      w1475 = "CANDTU.txt"
      n229 = xnode "匹配正则表达式"("输入字符串"=w1490, "正则表达式"="\\S*") -> ("所有匹配"=w1487:string)  [unwired: 4 in, 4 out]
      n230 = xnode "匹配正则表达式"("输入字符串"=w1492, "正则表达式"="\\S*") -> ("所有匹配"=w1488:string)  [unwired: 4 in, 4 out]
      n231 = Search and Replace String(replace all?=TRUE ("替换全部？(F)"), input string=w1504, search string="\n") -> (number of replacements=w1506:i32)  [unwired: 5 in, 3 out]
      n232 = Subtract(x=w1506, y=1) -> (x-y=w1503:i32)
      n233 = File/Directory Info(path=w1494) -> (last mod=w1498:timestamp)  [unwired: 1 in, 6 out]
      n234 = Fract/Exp String To Number(string=w1488) -> (number=w1485:dbl)  [unwired: 3 in, 1 out]
      n235 = Format Date/Time String(seconds (now)=w1498) -> (date/time string=w1496:string)  [unwired: 2 in]
      n236 = Fract/Exp String To Number(string=w1487) -> (number=w1486:dbl)  [unwired: 3 in, 1 out]
      n237 = Number To Decimal String(number=w1503) -> (decimal integer string=w1523:string)  [unwired: 1 in]
      n238 = Concatenate Strings(w1480, w1496, "\n") -> (w1495:string)
      n239 = Get File Size(file=w1494) -> (size (in bytes)=w1520:i64)  [unwired: 1 in, 2 out]
      n240 = Strip Path(path=w1494) -> (stripped path=w1500:path, name=w1531:string)
      n241 = Quotient & Remainder(x=w1520, y=w1517) -> (x-y*floor(x/y)=w1513:i64, floor(x/y)=w1519:i64)
      n242 = Subtract(x=w1486, y=w1485) -> (x-y=w1484:dbl)
      n243 = Quotient & Remainder(x=w1519, y=w1517) -> (x-y*floor(x/y)=w1515:i64, floor(x/y)=w1516:i64)
      n244 = Greater Than 0?(x=w1516) -> (x > 0?=w1518:bool)
      n245 = Path To String(path=w1500) -> (string=w1501:string)
      n246 = case shown="假" w1518 {
        tunnel: w1517 -> [w1771 w1781]
        tunnel: w1516 -> [_ w1779]
        tunnel: w1515 -> [w1769 w1782]
        tunnel: [w1774 w1777] -> w1514
        tunnel: w1513 -> [w1772 _]
        frame False {
          n247 = Divide(x=w1772, y=w1771) -> (x/y=w1770:dbl)
          n248 = Add(x=w1770, y=w1769) -> (x+y=w1768:dbl)
          n249 = Number To Fractional String(number=w1768, precision (6)=i16 2 ("精度(6)")) -> (F-format string=w1766:string)  [unwired: 2 in]
          n250 = Concatenate Strings(w1766, "KB" ("字符串")) -> (w1774:string)
        }
        frame True {
          n251 = Divide(x=w1782, y=w1781) -> (x/y=w1780:dbl)
          n252 = Add(x=w1779, y=w1780) -> (x+y=w1778:dbl)
          n253 = Number To Fractional String(number=w1778, precision (6)=i16 2 ("精度(6)")) -> (F-format string=w1776:string)  [unwired: 2 in]
          n254 = Concatenate Strings(w1776, "MB") -> (w1777:string)
        }
      }
      n255 = Number To Fractional String(number=w1484, precision (6)=i16 1 ("精度(6)")) -> (F-format string=w1482:string)  [unwired: 2 in]
      n256 = Concatenate Strings(w1476, w1475, "\n") -> (w1528:string)
      n257 = Concatenate Strings(w1479, w1501, "\n") -> (w1499:string)
      n258 = Concatenate Strings("总帧数：", w1523, "\n") -> (w1524:string)
      n259 = Concatenate Strings(w1477, w1514, "\n") -> (w1521:string)
      n260 = Concatenate Strings(w1478, w1531, "\n") -> (w1530:string)
      n261 = Concatenate Strings("首帧时间：", w1488, w1489, "\n") -> (w1512:string)
      n262 = Concatenate Strings("总时长：", w1482, " ms", "\n") -> (w1510:string)
      n263 = Concatenate Strings("末帧时间：", w1487, w1489, "\n") -> (w1511:string)
      n264 = Concatenate Strings(w1530, w1499, w1521, w1495, w1528, w1524, w1512, w1511, w1510) -> (w1509:string)
    }
  }
  "FileInfo" <- w40
  "文件类型" <- w39
  "路径输出" <- "file path (dialog if empty)"
